vi "Set Heater State.vi"(8 "error in (no error)":errorcluster, 10 "Heater State":T1, 11 "Thermal Chamber Controller In":refnum<class "Thermal Chamber Controller.lvclass">) -> (0 "error out":errorcluster, 3 "Thermal Chamber Controller Out":refnum<class "Thermal Chamber Controller.lvclass">)   [LabVIEW 2020, in "Thermal Chamber Controller.lvclass"]
uses:
  Thermal Chamber Controller.lvclass
  C:/Program Files (x86)/National Instruments/LabVIEW 2020/vi.lib/Astemes/Triarc Framework/Process/Process.lvclass
  Private/Heater State.ctl
  <vilib>/Astemes/Triarc Framework/Process/Process.lvclass/Process.ctl
  Thermal Chamber Controller.lvclass/Thermal Chamber Controller.ctl
  <vilib>/Utility/error.llb/Clear Errors.vi
  <vilib>/Astemes/Triarc Framework/Process/Private/SubVIs/Handle Debug Data.vi
  <vilib>/Utility/High Resolution Relative Seconds.vi
  <vilib>/Utility/error.llb/Error Cluster From Error Code.vi
  <vilib>/Astemes/Triarc Framework/Process/Process.lvclass
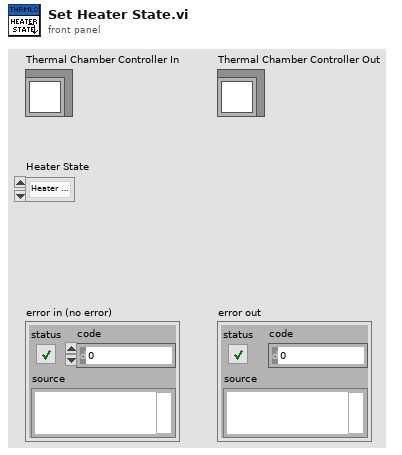
[diagram p1: front panel]
types:
  T1 = typedef "Thermal Chamber Controller.lvclass/Heater State.ctl" = enum16{"Heater Disabled", "Heater Enabled"}
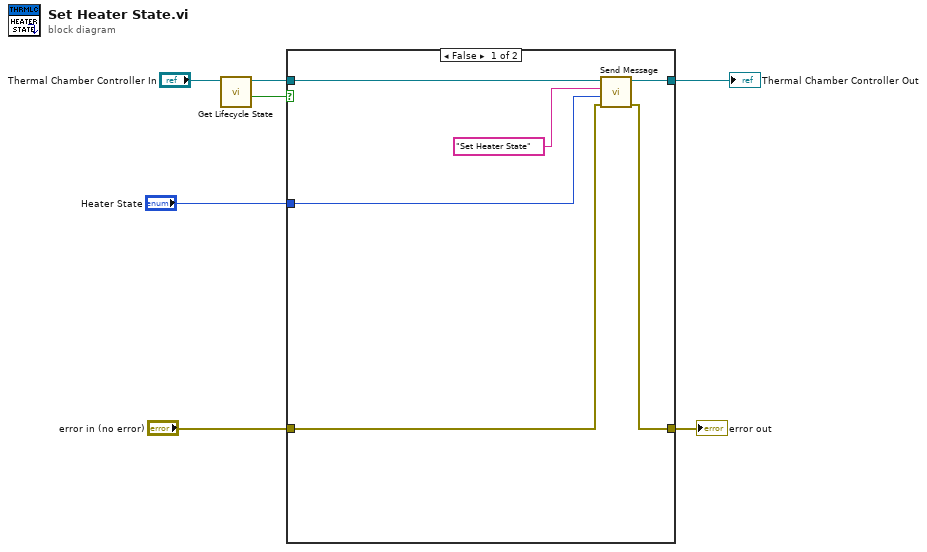
[diagram p0: block diagram]
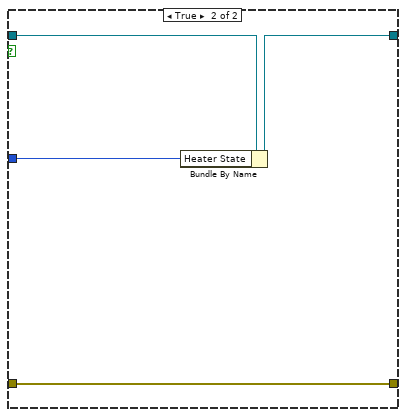
[diagram p2: hidden frame]
diagram:
  n1 = call <vilib>:"Get Lifecycle State.vi"("Process In"="Thermal Chamber Controller In") -> ("In Process Loop?"=w3:bool, "Process Out"=w6:refnum<class "Thermal Chamber Controller.lvclass">)  [unwired: 7 in, 2 out]
  n2 = case shown="False" w3 {
    tunnel: w6 -> [w13 w17]
    tunnel: [w12 w15] -> w5
    tunnel: "error in (no error)" -> [w8 w16]
    tunnel: [w9 w16] -> w4
    tunnel: "Heater State" -> [w11 w14]
    frame False {
      n3 = call <vilib>:"Send Message.vi"("error in (no error)"=w8, "Message Data"=w11, "Message"="Set Heater State" ("API Message"), "Process In"=w13) -> ("error out"=w9:errorcluster, "Process Out"=w12:refnum<class "Thermal Chamber Controller.lvclass">)  [unwired: 6 in]
    }
    frame True {
      n4 = Bundle By Name(cluster=w17, "Heater State"=w14) -> (w15:refnum<class "Thermal Chamber Controller.lvclass">)
    }
  }
  "error out" <- w4
  "Thermal Chamber Controller Out" <- w5
